vi "Add to Assembly Array.vi"(7 "Type":enum16{"To End", "To Front"}(ring), 8 "error in (no error)":errorcluster, 9 "Workspace In":refnum<class "Fixture.lvclass">, 10 "Routine In":refnum<class "Routine.lvclass">, 11 "Assembly Run in":refnum<class "Assembly Run.lvclass">) -> (0 "error out":errorcluster, 3 "Assembly Run out":refnum<class "Assembly Run.lvclass">)   [LabVIEW 2016, in "Assembly Run.lvclass"]
uses:
  Assembly Run.lvclass
  Routine/Routine.lvclass
  Workspace/Fixture.lvclass
  Assembly Run.lvclass/Assembly Run.ctl
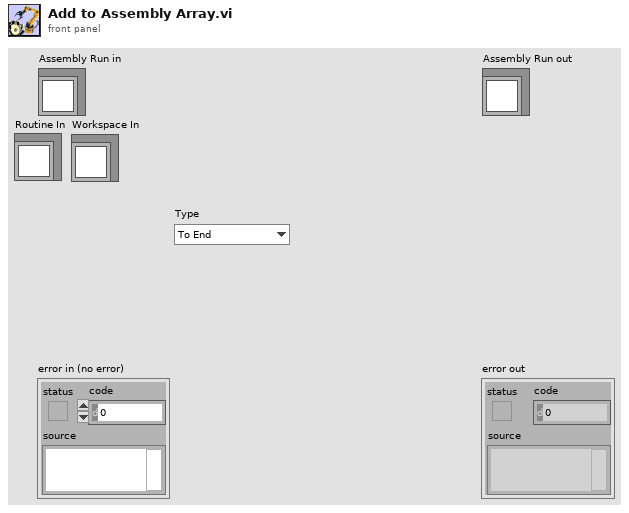
[diagram p1: front panel]
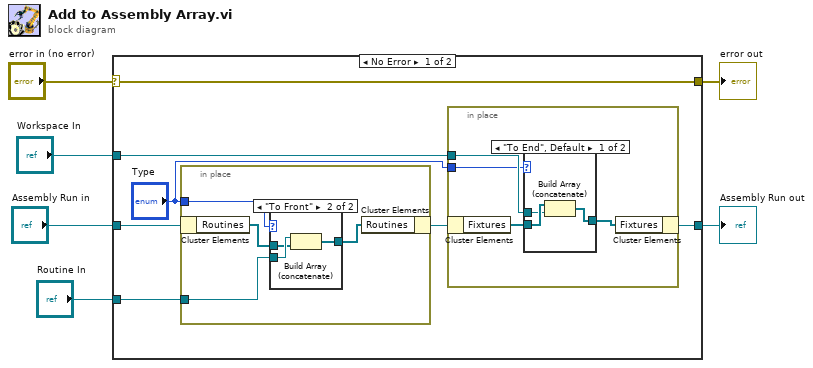
[diagram p0: block diagram]
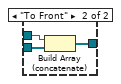
[diagram p2: hidden frame]
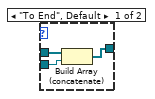
[diagram p3: hidden frame]
diagram:
  n1 = case shown="No Error" "error in (no error)" {
    selector: "error in (no error)" -> [w13 w35]
    tunnel: [w13 w35] -> w5
    tunnel: [w10 w34] -> w3
    tunnel: "Assembly Run in" -> [w11 w34]
    tunnel: "Routine In" -> [w9 _]
    tunnel: "Workspace In" -> [w8 _]
    frame No Error {
      n2 = in-place {
        in-place-border: w9 -> [w25]
        in-place-border: "Type" -> [w24]
        n3 = in-place-cluster #1(w11) -> ("Routines"=w26:refnum<class "Routine.lvclass">[])
        n4 = case shown="\"To Front\"" w24 {
          tunnel: [w30 w31] -> w27
          tunnel: w26 -> [w29 w32]
          tunnel: w25 -> [w28 w33]
          frame "To End", Default {
            n5 = Build Array (concatenate)(w29, w28) -> (w30:refnum<class "Routine.lvclass">[])
          }
          frame "To Front" {
            n6 = Build Array (concatenate)(w33, w32) -> (w31:refnum<class "Routine.lvclass">[])
          }
        }
        n7 = in-place-cluster #1("Routines"=w27) -> (w12:refnum<class "Assembly Run.lvclass">)
      }
      n8 = in-place {
        in-place-border: w8 -> [w16]
        in-place-border: "Type" -> [w14]
        n9 = in-place-cluster #2(w12) -> ("Fixtures"=w17:refnum<class "Fixture.lvclass">[])
        n10 = case shown="\"To End\", Default" w14 {
          tunnel: w17 -> [w20 w22]
          tunnel: w16 -> [w19 w23]
          tunnel: [w18 w21] -> w15
          frame "To End", Default {
            n11 = Build Array (concatenate)(w20, w19) -> (w18:refnum<class "Fixture.lvclass">[])
          }
          frame "To Front" {
            n12 = Build Array (concatenate)(w23, w22) -> (w21:refnum<class "Fixture.lvclass">[])
          }
        }
        n13 = in-place-cluster #2("Fixtures"=w15) -> (w10:refnum<class "Assembly Run.lvclass">)
      }
    }
    frame Error {
    }
  }
  "error out" <- w5
  "Assembly Run out" <- w3
